vi "fpga_library.vi"() -> ()   [LabVIEW 2014]
uses:
  <vilib>/rvi/Emulation/niFpgaGetClockAttributes.vi
  <vilib>/rvi/Emulation/niFpgaSctlEmulationGetInTimedLoop.vi
  <vilib>/rvi/Emulation/niFpgaEmulationReportErrorSimple.vi
  <vilib>/rvi/interface/RandomDataEmulation/niFpgaRandomDataHandleErrors.vi
  <vilib>/rvi/eio/common/nirviEmuTemplateMethod_errors.vi
  <vilib>/rvi/Emulation/niFpgaCriticalErrorInLSC.vi
  <vilib>/rvi/DataTransferAndStorage/Container/XNode/niFpgaContainer.xnode
  <vilib>/rvi/interface/RandomDataEmulation/nirviRandomDataFpgaReadWriteTemplate.vi
  <vilib>/eio/EIONode/EIONode.xnode
panel:
  in  "Count(Ticks)":u32=907
  out "Actual Period (tics)":u32
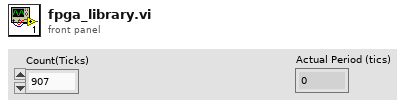
[diagram p1: front panel]
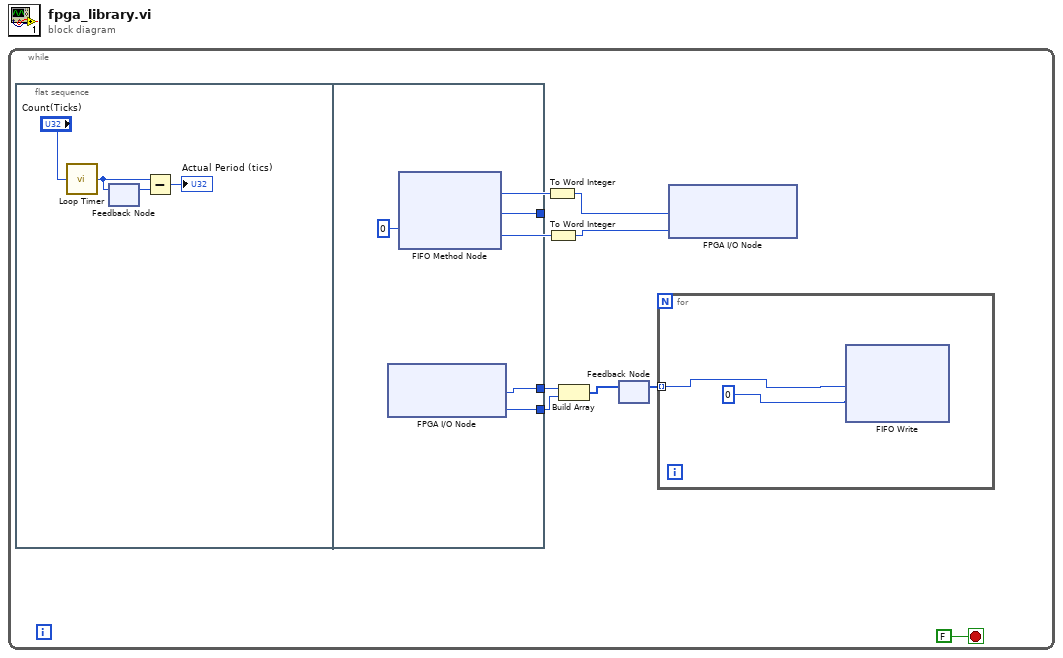
[diagram p0: block diagram]
diagram:
  n1 = while {
    stop <- FALSE stop-if-true
    n2 = flat-sequence {
      tunnel: [w18] -> w5
      tunnel: [w16] -> w3
      tunnel: [w15] -> w2
      frame #0 {
        n3 = call "Loop Timer"("Count(Ticks)"="Count(Ticks)") -> ("Tick Count(Ticks)"=w13:u32)
        n4 = feedback #1() -> (w12:u32)  [unwired: 1 in]
        n5 = feedback-in #1(w13) -> ()
        n6 = Subtract(x=w13, y=w12) -> (x-y=→"Actual Period (tics)":u32)
      }
      frame #1 {
        n7 = xnode "FPGA I/O Node"() -> ("AudioIn/Left"=w16:i16, "AudioIn/Right"=w15:i16)  [unwired: 2 in, 2 out]
        n8 = xnode ("FIFO Method Node")("Timeout"=0) -> ("Element"=w18:u32)  [unwired: 1 in, 2 out]
      }
    }
    n9 = To Word Integer(number=w5) -> (16bit integer=w6:i16)
    n10 = To Word Integer(number=w5) -> (16bit integer=w7:i16)
    n11 = Build Array(w3, w2) -> (w1:i16[])
    n12 = feedback #2() -> (w4:i16[])  [unwired: 1 in]
    n13 = feedback-in #2(w1) -> ()
    n14 = for {
      tunnel: w4 -> [w10] mode=indexing
      n15 = xnode ("FIFO Write")("Element"=w10, "Timeout"=0) -> ()  [unwired: 1 in, 2 out]
    }
    n16 = xnode "FPGA I/O Node"("AudioOut/Left"=w6, "AudioOut/Right"=w7) -> ()  [unwired: 2 in, 2 out]
  }
